vi "input.vi"(8 "error in":errorcluster, 10 "data table in":T1, 11 "EthernetIP runtime in":refnum<class "EIP Tags Runtime.lvclass">) -> (0 "error out":errorcluster, 2 "data table out":T1, 3 "EthernetIP runtime out":refnum<class "EIP Tags Runtime.lvclass">)   [LabVIEW 2013, in "EIP Tags Runtime.lvclass"]
doc: "Provides an interface for reading data from a module at runtime. While this interface performs no operations, a child should provide an override which may read from any open sessions, references, or interfaces."
uses:
  EIP Tags Runtime.lvclass
  <vilib>/NI/Tag Bus/table/data table.ctl
  EIP Tags Runtime.lvclass/EIP Tags Runtime.ctl
  <vilib>/NI/Tag Bus/table/data polymorphs/write many/write I8s.vi
  <vilib>/NI/Tag Bus/table/data polymorphs/write one/write Array of I8.vi
  <vilib>/NI/Tag Bus/table/data polymorphs/write many/write I16s.vi
  <vilib>/NI/Tag Bus/table/data polymorphs/write one/write Array of I16.vi
  <vilib>/NI/Tag Bus/table/data polymorphs/write many/write I32s.vi
  <vilib>/NI/Tag Bus/table/data polymorphs/write one/write Array of I32.vi
  <vilib>/NI/Tag Bus/table/data polymorphs/write many/write Singles.vi
  <vilib>/NI/Tag Bus/table/data polymorphs/write one/write Array of Single.vi
  <vilib>/NI/Tag Bus/table/data polymorphs/write many/write Booleans.vi
  <vilib>/NI/Tag Bus/table/data polymorphs/write one/write Array of Boolean.vi
  <vilib>/NI/Tag Bus/table/data polymorphs/write one/write String.vi
  <vilib>/ethernetip/ethernetip.llb/EthernetIP Tag Read SINT.vi
  <vilib>/ethernetip/ethernetip.llb/EthernetIP Tag Read INT.vi
  <vilib>/ethernetip/ethernetip.llb/EthernetIP Tag Read DINT.vi
  <vilib>/ethernetip/ethernetip.llb/EthernetIP Tag Read REAL.vi
  <vilib>/ethernetip/ethernetip.llb/EthernetIP Tag Read BOOL.vi
  <vilib>/ethernetip/ethernetip.llb/EthernetIP Tag Read STRING.vi
  <vilib>/ethernetip/ethernetip.lvlib
  <vilib>/NI/Tag Bus/table/data table.lvlib
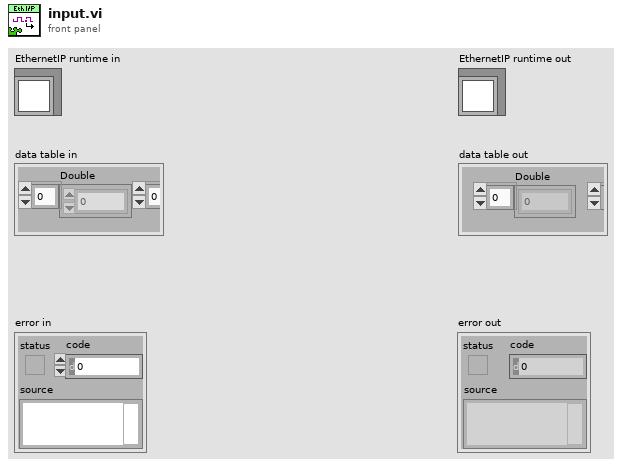
[diagram p1: front panel]
types:
  T1 = typedef "tag bus.lvlib/data table.lvlib/data table.ctl" = cluster{"Double":dbl[], "Single":sgl[], "I64":i64[], "I32":i32[], "I16":i16[], "I8":i8[], "U64":u64[], "U32":u32[], "U16":u16[], "U8":u8[], "Boolean":bool[], "String":string[], "Array of Double":cluster{"DBL Array":dbl[]}[], "Array of Single":cluster{"SGL Array":sgl[]}[], "Array of I64":cluster{"I64 Array":i64[]}[], "Array of I32":cluster{"I32 Array":i32[]}[], "Array of I16":cluster{"I16 Array":i16[]}[], "Array of I8":cluster{"I8 Array":i8[]}[], "Array of U64":cluster{"U64 Array":u64[]}[], "Array of U32":cluster{"U32 Array":u32[]}[], "Array of U16":cluster{"U16 Array":u16[]}[], "Array of U8":cluster{"U8 Array":u8[]}[], "Array of Boolean":cluster{"Boolean Array":bool[]}[], "Array of String":cluster{"String Array":string[]}[]}
  T2 = typedef "ethernetip.lvlib/ethernetip.ctl" = refnum<k21>
  T3 = typedef "EIP Tags Runtime.lvclass/eip tag spec.ctl" = cluster{"eip tag types":T4, "Network Path":string, "Tag Name":string, "Number of Elements":u32, "data indices":i32[], "tag bus indices":i32[], "array tbtag":bool}
  T4 = typedef "EIP Tags Configuration.lvclass/eip tag types.ctl" = enum16{"SINT", "INT", "DINT", "REAL", "BOOL", "STRING"}
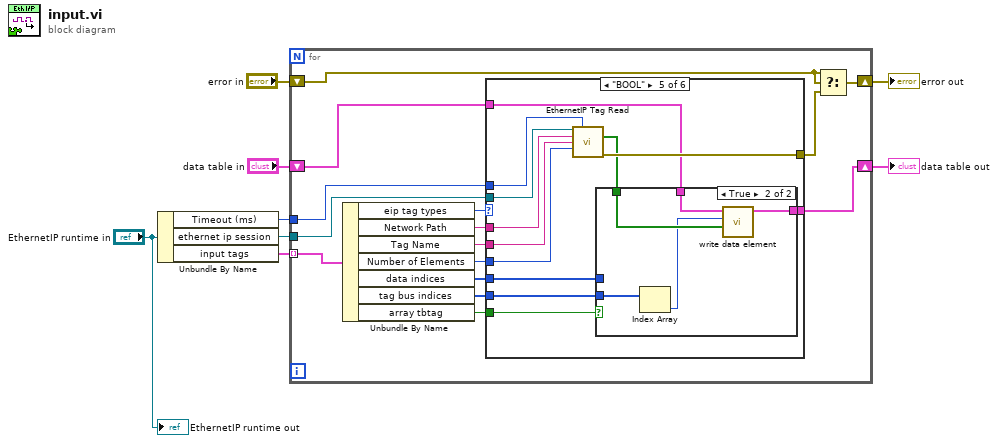
[diagram p0: block diagram]
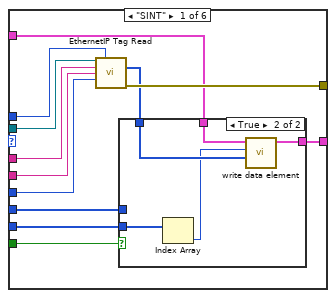
[diagram p2: hidden frame]
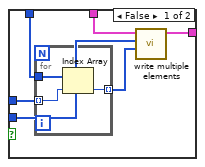
[diagram p3: hidden frame]
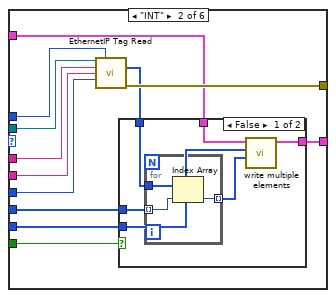
[diagram p4: hidden frame]
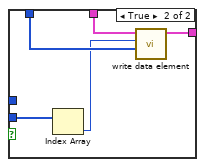
[diagram p5: hidden frame]
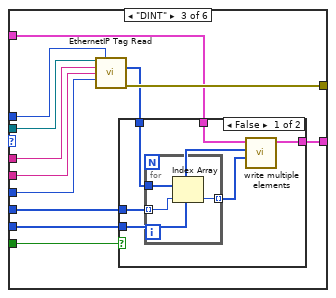
[diagram p6: hidden frame]
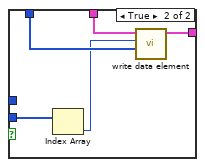
[diagram p7: hidden frame]
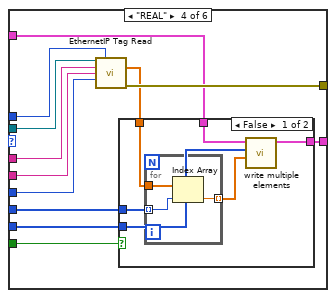
[diagram p8: hidden frame]
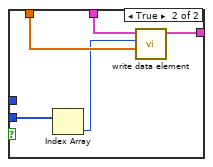
[diagram p9: hidden frame]
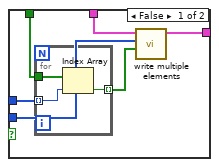
[diagram p10: hidden frame]
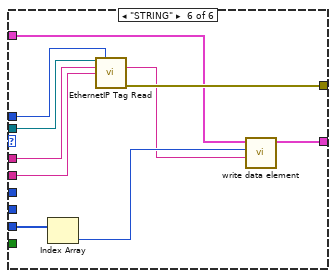
[diagram p11: hidden frame]
diagram:
  n1 = Unbundle By Name("EthernetIP runtime in") -> ("Timeout (ms)"=w1:i32, "ethernet ip session"=w7:T2, "input tags"=w4:T3[])
  n2 = for {
    tunnel: w7 -> [w19]
    shift-right: [w22] -> w5
    shift-left: "error in" -> [w23]
    tunnel: w4 -> [w21] mode=indexing
    shift-right: [w15] -> w2
    shift-left: "data table in" -> [w16]
    tunnel: w1 -> [w18]
    n3 = Unbundle By Name(w21) -> ("eip tag types"=w20:T4, "Network Path"=w14:string, "Tag Name"=w13:string, "Number of Elements"=w12:u32, "data indices"=w11:i32[], "tag bus indices"=w10:i32[], "array tbtag"=w9:bool)
    n4 = case shown="\"BOOL\"" w20 {
      tunnel: w19 -> [w35 w61 w87 w113 w139 w163]
      tunnel: w18 -> [w34 w60 w86 w112 w138 w162]
      tunnel: [w33 w59 w85 w111 w137 w161] -> w17
      tunnel: w16 -> [w26 w52 w78 w104 w130 w157]
      tunnel: [w27 w53 w79 w105 w131 w158] -> w15
      tunnel: w14 -> [w32 w58 w84 w110 w136 w160]
      tunnel: w13 -> [w31 w57 w83 w109 w135 w159]
      tunnel: w12 -> [w30 w56 w82 w108 w134 _]
      tunnel: w11 -> [w28 w54 w80 w106 w132 _]
      tunnel: w10 -> [w25 w51 w77 w103 w129 w156]
      tunnel: w9 -> [w24 w50 w76 w102 w128 _]
      frame "SINT" {
        n5 = call-poly <vilib>:"EthernetIP Tag Read.vi"("Session in"=w35, "Timeout (ms)"=w34, "Network Path"=w32, "Tag Name"=w31, "Number of Elements"=w30) -> ("Data"=w29:i8[], "error out"=w33:errorcluster)  [unwired: 8 in, 1 out]
        n6 = case shown="True" w24 {
          tunnel: w29 -> [w41 w47]
          tunnel: w28 -> [w40 _]
          tunnel: [w39 w49] -> w27
          tunnel: w26 -> [w38 w48]
          tunnel: w25 -> [w36 w46]
          frame False {
            n7 = for {
              tunnel: w41 -> [w44]
              tunnel: w40 -> [w43] mode=indexing
              tunnel: [w42] -> w37 mode=indexing
              n8 = Index Array(array=w44, index=w43) -> (element=w42:i8)
            }
            n9 = call-poly <vilib>:"write multiple elements.vi"("values"=w37, "indices"=w36, "data table in"=w38) -> ("data table out"=w39:T1)  [unwired: 8 in]
          }
          frame True {
            n10 = Index Array(array=w46) -> (element=w45:i32)  [unwired: 1 in]
            n11 = call-poly <vilib>:"write data element.vi"("value"=w47, "index"=w45, "data table in"=w48) -> ("data table out"=w49:T1)  [unwired: 8 in]
          }
        }
      }
      frame "INT" {
        n12 = call-poly <vilib>:"EthernetIP Tag Read.vi"("Session in"=w61, "Timeout (ms)"=w60, "Network Path"=w58, "Tag Name"=w57, "Number of Elements"=w56) -> ("Data"=w55:i16[], "error out"=w59:errorcluster)  [unwired: 8 in, 1 out]
        n13 = case shown="False" w50 {
          tunnel: w55 -> [w67 w73]
          tunnel: w54 -> [w66 _]
          tunnel: [w65 w75] -> w53
          tunnel: w52 -> [w64 w74]
          tunnel: w51 -> [w62 w72]
          frame False {
            n14 = for {
              tunnel: w67 -> [w70]
              tunnel: w66 -> [w69] mode=indexing
              tunnel: [w68] -> w63 mode=indexing
              n15 = Index Array(array=w70, index=w69) -> (element=w68:i16)
            }
            n16 = call-poly <vilib>:"write multiple elements.vi"("values"=w63, "indices"=w62, "data table in"=w64) -> ("data table out"=w65:T1)  [unwired: 8 in]
          }
          frame True {
            n17 = Index Array(array=w72) -> (element=w71:i32)  [unwired: 1 in]
            n18 = call-poly <vilib>:"write data element.vi"("value"=w73, "index"=w71, "data table in"=w74) -> ("data table out"=w75:T1)  [unwired: 8 in]
          }
        }
      }
      frame "DINT" {
        n19 = call-poly <vilib>:"EthernetIP Tag Read.vi"("Session in"=w87, "Timeout (ms)"=w86, "Network Path"=w84, "Tag Name"=w83, "Number of Elements"=w82) -> ("Data"=w81:i32[], "error out"=w85:errorcluster)  [unwired: 8 in, 1 out]
        n20 = case shown="False" w76 {
          tunnel: w81 -> [w93 w99]
          tunnel: w80 -> [w92 _]
          tunnel: [w91 w101] -> w79
          tunnel: w78 -> [w90 w100]
          tunnel: w77 -> [w88 w98]
          frame False {
            n21 = for {
              tunnel: w93 -> [w96]
              tunnel: w92 -> [w95] mode=indexing
              tunnel: [w94] -> w89 mode=indexing
              n22 = Index Array(array=w96, index=w95) -> (element=w94:i32)
            }
            n23 = call-poly <vilib>:"write multiple elements.vi"("values"=w89, "indices"=w88, "data table in"=w90) -> ("data table out"=w91:T1)  [unwired: 8 in]
          }
          frame True {
            n24 = Index Array(array=w98) -> (element=w97:i32)  [unwired: 1 in]
            n25 = call-poly <vilib>:"write data element.vi"("value"=w99, "index"=w97, "data table in"=w100) -> ("data table out"=w101:T1)  [unwired: 8 in]
          }
        }
      }
      frame "REAL" {
        n26 = call-poly <vilib>:"EthernetIP Tag Read.vi"("Session in"=w113, "Timeout (ms)"=w112, "Network Path"=w110, "Tag Name"=w109, "Number of Elements"=w108) -> ("Data"=w107:sgl[], "error out"=w111:errorcluster)  [unwired: 8 in, 1 out]
        n27 = case shown="False" w102 {
          tunnel: w107 -> [w119 w125]
          tunnel: w106 -> [w118 _]
          tunnel: [w117 w127] -> w105
          tunnel: w104 -> [w116 w126]
          tunnel: w103 -> [w114 w124]
          frame False {
            n28 = for {
              tunnel: w119 -> [w122]
              tunnel: w118 -> [w121] mode=indexing
              tunnel: [w120] -> w115 mode=indexing
              n29 = Index Array(array=w122, index=w121) -> (element=w120:sgl)
            }
            n30 = call-poly <vilib>:"write multiple elements.vi"("values"=w115, "indices"=w114, "data table in"=w116) -> ("data table out"=w117:T1)  [unwired: 8 in]
          }
          frame True {
            n31 = Index Array(array=w124) -> (element=w123:i32)  [unwired: 1 in]
            n32 = call-poly <vilib>:"write data element.vi"("value"=w125, "index"=w123, "data table in"=w126) -> ("data table out"=w127:T1)  [unwired: 8 in]
          }
        }
      }
      frame "BOOL" {
        n33 = call-poly <vilib>:"EthernetIP Tag Read.vi"("Session in"=w139, "Timeout (ms)"=w138, "Network Path"=w136, "Tag Name"=w135, "Number of Elements"=w134) -> ("Data"=w133:bool[], "error out"=w137:errorcluster)  [unwired: 8 in, 1 out]
        n34 = case shown="True" w128 {
          tunnel: w133 -> [w145 w151]
          tunnel: w132 -> [w144 _]
          tunnel: [w143 w153] -> w131
          tunnel: w130 -> [w142 w152]
          tunnel: w129 -> [w140 w150]
          frame False {
            n35 = for {
              tunnel: w145 -> [w148]
              tunnel: w144 -> [w147] mode=indexing
              tunnel: [w146] -> w141 mode=indexing
              n36 = Index Array(array=w148, index=w147) -> (element=w146:bool)
            }
            n37 = call-poly <vilib>:"write multiple elements.vi"("values"=w141, "indices"=w140, "data table in"=w142) -> ("data table out"=w143:T1)  [unwired: 8 in]
          }
          frame True {
            n38 = Index Array(array=w150) -> (element=w149:i32)  [unwired: 1 in]
            n39 = call-poly <vilib>:"write data element.vi"("value"=w151, "index"=w149, "data table in"=w152) -> ("data table out"=w153:T1)  [unwired: 8 in]
          }
        }
      }
      frame "STRING" {
        n40 = Index Array(array=w156) -> (element=w155:i32)  [unwired: 1 in]
        n41 = call-poly <vilib>:"EthernetIP Tag Read.vi"("Session in"=w163, "Timeout (ms)"=w162, "Network Path"=w160, "Tag Name"=w159) -> ("Data"=w154:string, "error out"=w161:errorcluster)  [unwired: 9 in, 1 out]
        n42 = call-poly <vilib>:"write data element.vi"("value"=w154, "index"=w155, "data table in"=w157) -> ("data table out"=w158:T1)  [unwired: 8 in]
      }
    }
    n43 = Select(t=w23, s=w23, f=w17) -> (s? t:f=w22:errorcluster)
  }
  "error out" <- w5
  "data table out" <- w2
  "EthernetIP runtime out" <- "EthernetIP runtime in"
